vi "API_GetUserName.vi"(2 "error in (no error)":errorcluster) -> (0 "error out":errorcluster, 1 "User Name":string)   [LabVIEW 2012, in "API.lvlib"]
doc: "Uses an API call to retrieve the user name"
uses:
  API.lvlib
  advapi32.dll
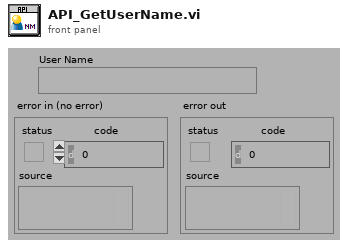
[diagram p1: front panel]
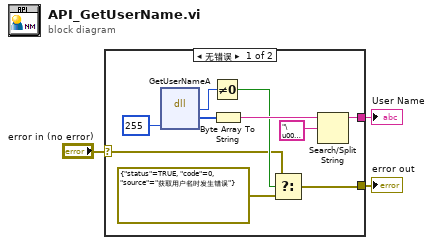
[diagram p0: block diagram]
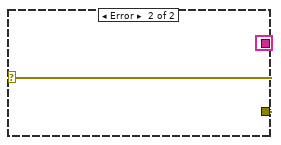
[diagram p2: hidden frame]
diagram:
  n1 = case shown="无错误" "error in (no error)" {
    selector: "error in (no error)" -> [w4 w14]
    tunnel: [w10 "" ("string")] -> w3
    tunnel: [w7 w14] -> w2
    frame No Error {
      n2 = dll-call lib="advapi32.dll" fn="GetUserNameA"("nSize"=u32 255) -> ("返回类型"=w9:u8, "lpBuffer"=w13:u8[])  [unwired: 5 in, 2 out]
      n3 = Not Equal To 0?(x=w9) -> (x != 0?=w8:bool)
      n4 = Byte Array To String(unsigned byte array=w13) -> (string=w12:string)
      n5 = Select(t=w4, s=w8, f=errorcluster {"status"=TRUE, "code"=0, "source"="获取用户名时发生错误"}) -> (s? t:f=w7:errorcluster)
      n6 = Search/Split String(string=w12, search string/char (-)="\u0000" ("regular expression")) -> (substring before match=w10:string)  [unwired: 1 in, 2 out]
    }
    frame Error {
    }
  }
  "User Name" <- w3
  "error out" <- w2
